vi "MEMR-Dispose of Data Files.vi"(0 "State":T1, 11 "error in (no error)":errorcluster) -> (4 "file pattern":path, 15 "error out":errorcluster)   [LabVIEW 2020]
uses:
  Typedefs/MEMR-Analysis State.ctl
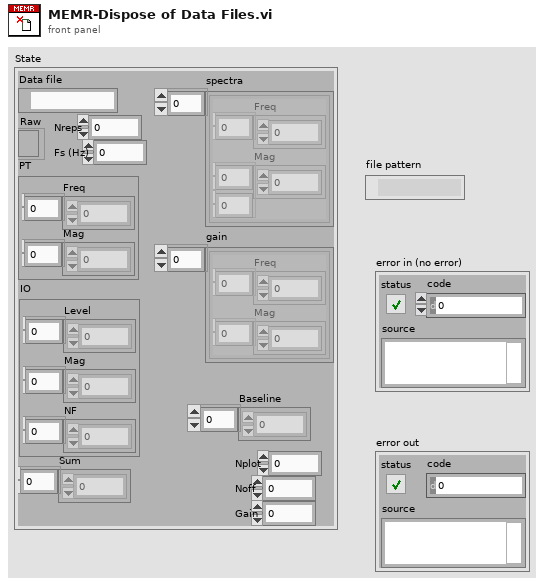
[diagram p1: front panel]
types:
  T1 = typedef "MEMR-Analysis State.ctl" = cluster{"Data file":path, "Raw":refnum<file>, "PT":cluster{"Freq":dbl[], "Mag":dbl[]}, "IO":cluster{"Level":dbl[], "Mag":dbl[], "NF":dbl[]}, "Nreps":i32, "Fs (Hz)":dbl, "Sum":dbl[], "Nplot":i32, "Noff":i32, "Gain":dbl, "spectra":cluster{"Freq":dbl[], "Mag":dbl[][]}[], "gain":cluster{"Freq":dbl[], "Mag":dbl[]}[], "Baseline":dbl[]}
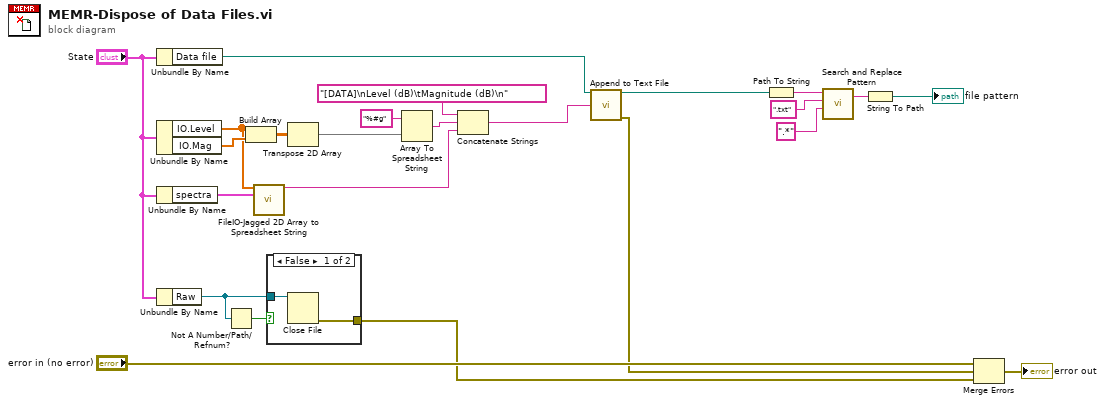
[diagram p0: block diagram]
diagram:
  n1 = Unbundle By Name("State") -> ("Data file"=w19:path)
  n2 = Unbundle By Name("State") -> ("IO.Level"=w3:dbl[], "IO.Mag"=w24:dbl[])
  n3 = Unbundle By Name("State") -> ("spectra"=w2:cluster{"Freq":dbl[], "Mag":dbl[][]}[])
  n4 = Unbundle By Name("State") -> ("Raw"=w12:refnum<file>)
  n5 = Not A Number/Path/Refnum?(number/path/refnum=w12) -> (NaN/Path/Refnum?=w11:bool)
  n6 = Build Array(w3, w24) -> (w23:dbl[][])
  n7 = call "FileIO-Jagged 2D Array to Spreadsheet String.vi"("seqVals"=w3, "spectra"=w2) -> ("spreadsheet string"=w1:string)  [unwired: 13 in]
  n8 = case shown="False" w11 {
    tunnel: w12 -> [w26 _]
    tunnel: [w25 _] -> w7
    frame False {
      n9 = Close File(refnum=w26) -> (error out=w25:errorcluster)  [unwired: 1 in, 1 out]
    }
    frame True {
    }
  }
  n10 = Transpose 2D Array(2D array=w23) -> (transposed array=w5:dbl[][])
  n11 = Array To Spreadsheet String(array=w5, 3:"%#g" ("format string")) -> (spreadsheet string=w21:string)  [unwired: 1 in]
  n12 = Concatenate Strings("[DATA]\nLevel (dB)\tMagnitude (dB)\n" ("string"), w21, w1) -> (w18:string)
  n13 = call "Append to Text File.vi"("file path"=w19, "text"=w18) -> ("file path out"=w17:path, "error out"=w8:errorcluster)  [unwired: 12 in]
  n14 = Path To String(path=w17) -> (string=w16:string)
  n15 = call <vilib>:"Search and Replace Pattern.vi"("string"=w16, "regular expression (\"\")"=".txt" ("regular expression (\"\")"), "replace string (\"\")"=".*" ("regular expression (\"\")")) -> ("result string"=w13:string)  [unwired: 2 in, 1 out]
  n16 = String To Path(string=w13) -> (path=→"file pattern":path)
  n17 = Merge Errors("error in (no error)", w8, w7) -> (→"error out":errorcluster)
